vi "Add Script.vi"(8 "error in":errorcluster, 10 "Script UI Ctrl Ref":T2, 11 "Script Meas Config Ctrl Ref":T1) -> (0 "error out":errorcluster)   [LabVIEW 2025, in "Fgen Script Mode UI.lvlib"]
uses:
  Fgen Script Mode UI.lvlib
  Typedef/Script UI Ctrl Ref.ctl
  Typedef/Script Meas Config Ctrl Ref.ctl
panel:
  in  "Cancel":bool
  in  "OK":bool
  in  "New Script Name":string
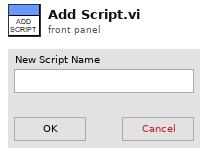
[diagram p1: front panel]
types:
  T1 = typedef "Fgen Script Mode UI.lvlib/Script Meas Config Ctrl Ref.ctl" = cluster{"Scripts Ref":refnum<vi>, "Script Names Ref":refnum<vi>, "Selected Script":refnum<vi>}
  T2 = typedef "Fgen Script Mode UI.lvlib/Script UI Ctrl Ref.ctl" = cluster{"Script Body Ref":refnum<vi>, "Selected Script (Ring) Ref":refnum<vi>, "Script Header Ref":refnum<vi>}
  T3 = enum16{"Cancelled", "Valid Scipt Name", "Invalid Script Name", "Conflict Script Name"}
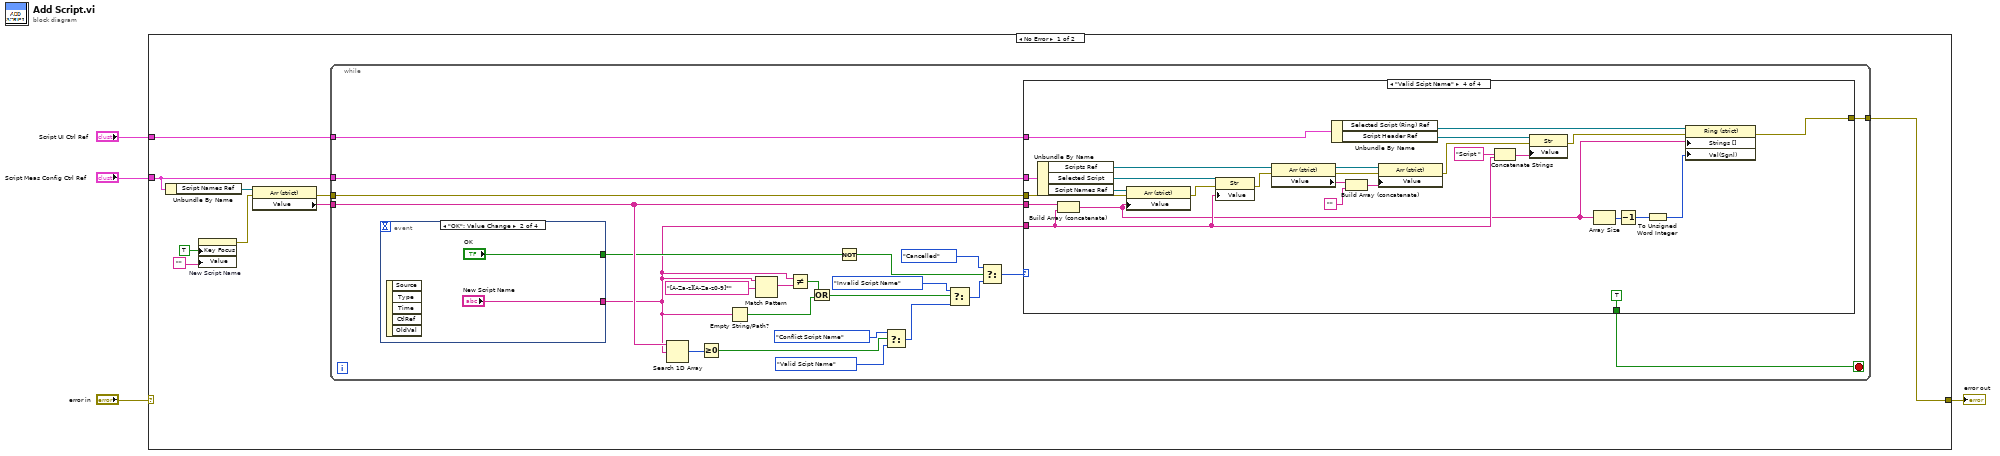
[diagram p0: block diagram]
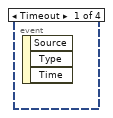
[diagram p2: hidden frame]
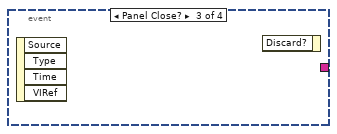
[diagram p3: hidden frame]
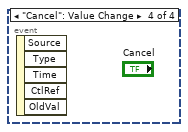
[diagram p4: hidden frame]
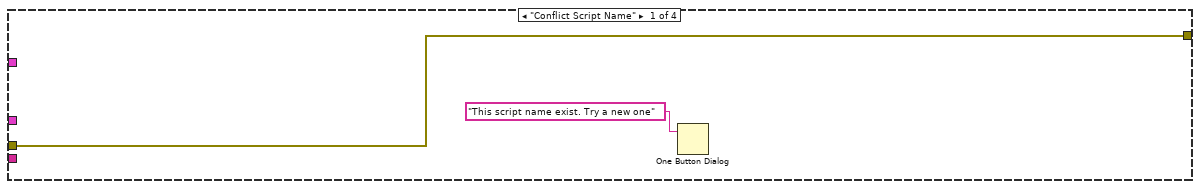
[diagram p5: hidden frame]
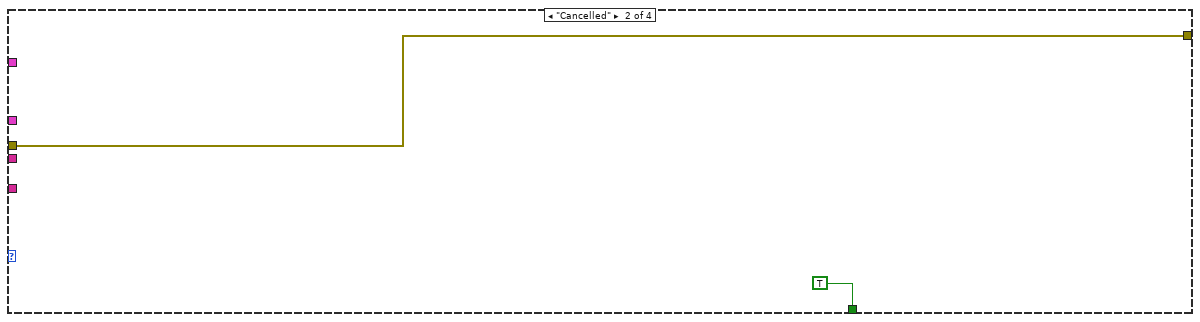
[diagram p6: hidden frame]
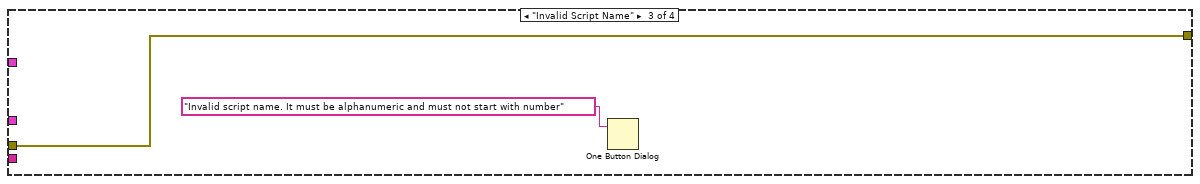
[diagram p7: hidden frame]
diagram:
  n1 = case shown="No Error" "error in" {
    selector: "error in" -> [_ w72]
    tunnel: [w9 w72] -> w3
    tunnel: "Script Meas Config Ctrl Ref" -> [w10 _]
    tunnel: "Script UI Ctrl Ref" -> [w11 _]
    frame No Error {
      n2 = Unbundle By Name(w10) -> ("Script Names Ref"=w13:refnum<vi>)
      n3 = property on="New Script Name" class="Str"("Key Focus"=TRUE, "Value"="") -> (error out=w6:errorcluster)  [unwired: 2 in, 1 out]
      n4 = property class="Arr (strict)"(reference=w13, error in=w6) -> (error out=w8:errorcluster, "Value"=w12:string[])  [unwired: 1 out]
      n5 = while {
        tunnel: w12 -> [w35]
        tunnel: w11 -> [w34]
        tunnel: w10 -> [w33]
        tunnel: [w19] -> w9
        tunnel: w8 -> [w18]
        stop <- w27 stop-if-true
        n6 = event shown="[1] \"OK\": Value Change" {
          selector: _ -> [_ _ _ _]
          dyn-events: _ -> [_ _ _ _]
          timeout: _ -> [_ _ _ _]
          tunnel: [_ "New Script Name" _ _] -> w15
          tunnel: [_ "OK" _ _] -> w17
          event Timeout {
            n7 = event-data() -> ()  [unwired: 1 in, 3 out]
          }
          event "OK": Value Change {
            n8 = event-data() -> ()  [unwired: 1 in, 5 out]
          }
          event Panel Close? {
            n9 = event-data() -> ()  [unwired: 1 in, 4 out]
            n10 = event-data() -> ()  [unwired: 2 in, 1 out]
          }
          event "Cancel": Value Change {
            n11 = event-data() -> ()  [unwired: 1 in, 5 out]
          }
        }
        n12 = Search 1D Array(1D array=w35, element=w15) -> (index of element=w36:i32)  [unwired: 1 in]
        n13 = Greater Or Equal To 0?(x=w36) -> (x >= 0?=w29:bool)
        n14 = Empty String/Path?(string/path=w15) -> (empty?=w14:bool)
        n15 = Match Pattern(string=w15, regular expression="[A-Za-z][A-Za-z0-9]*") -> (match substring=w31:string)  [unwired: 1 in, 3 out]
        n16 = Not Equal?(x=w15, y=w31) -> (x != y?=w30:bool)
        n17 = Or(x=w30, y=w14) -> (x .or. y?=w16:bool)
        n18 = Not(x=w17) -> (.not. x?=w25:bool)
        n19 = Select(t=T3."Conflict Script Name", s=w29, f=T3."Valid Scipt Name") -> (s? t:f=w28:T3)
        n20 = Select(t=T3."Invalid Script Name", s=w16, f=w28) -> (s? t:f=w26:T3)
        n21 = Select(t=T3."Cancelled", s=w25, f=w26) -> (s? t:f=w20:T3)
        n22 = case shown="\"Valid Scipt Name\"" w20 {
          tunnel: w35 -> [_ _ _ w71]
          tunnel: w15 -> [_ _ _ w67]
          tunnel: w34 -> [_ _ _ w70]
          tunnel: w33 -> [_ _ _ w55]
          tunnel: [_ TRUE _ TRUE] -> w27
          tunnel: [w39 w41 w43 w46] -> w19
          tunnel: w18 -> [w39 w41 w43 w45]
          frame "Conflict Script Name" {
            n23 = One Button Dialog(message="This script name exist. Try a new one") -> ()  [unwired: 1 in, 1 out]
          }
          frame "Cancelled" {
          }
          frame "Invalid Script Name" {
            n24 = One Button Dialog(message="Invalid script name. It must be alphanumeric and must not start with number") -> ()  [unwired: 1 in, 1 out]
          }
          frame "Valid Scipt Name" {
            n25 = Unbundle By Name(w55) -> ("Scripts Ref"=w53:refnum<vi>, "Selected Script"=w54:refnum<vi>, "Script Names Ref"=w56:refnum<vi>)
            n26 = Build Array (concatenate)(w71, w67) -> (w64:string[])
            n27 = property class="Arr (strict)"(reference=w56, error in=w45, "Value"=w64) -> (error out=w51:errorcluster)  [unwired: 1 out]
            n28 = property class="Str"(reference=w54, error in=w51, "Value"=w67) -> (error out=w50:errorcluster)  [unwired: 1 out]
            n29 = property class="Arr (strict)"(reference=w53, error in=w50) -> (reference out=w60:refnum<vi>, error out=w49:errorcluster, "Value"=w59:string[])
            n30 = Unbundle By Name(w70) -> ("Selected Script (Ring) Ref"=w65:refnum<vi>, "Script Header Ref"=w69:refnum<vi>)
            n31 = Build Array (concatenate)(w59, "") -> (w58:string[])
            n32 = property class="Arr (strict)"(reference=w60, error in=w49, "Value"=w58) -> (error out=w48:errorcluster)  [unwired: 1 out]
            n33 = Concatenate Strings("Script " ("format string"), w67) -> (w66:string)
            n34 = property class="Str"(reference=w69, error in=w48, "Value"=w66) -> (error out=w47:errorcluster)  [unwired: 1 out]
            n35 = Array Size(array=w64) -> (size(s)=w63:i32)
            n36 = Decrement(x=w63) -> (x-1=w62:i32)
            n37 = To Unsigned Word Integer(number=w62) -> (unsigned 16bit integer=w61:u16)
            n38 = property class="Ring (strict)"(reference=w65, error in=w47, "Strings []"=w64, "Val(Sgnl)"=w61) -> (error out=w46:errorcluster)  [unwired: 1 out]
          }
        }
      }
    }
    frame Error {
    }
  }
  "error out" <- w3
